vi "getValue.vi"(8 "error in (no error)":errorcluster, 11 "tBSONBoolean in":refnum<class "tBSONBoolean.lvclass">) -> (0 "error out":errorcluster, 2 "Value":bool, 3 "tBSONBoolean out":refnum<class "tBSONBoolean.lvclass">)   [LabVIEW 2013, in "BSON.lvlib" / "tBSONBoolean.lvclass"]
uses:
  tBSONBoolean.lvclass
  tBSONBoolean.lvclass/tBSONBoolean.ctl
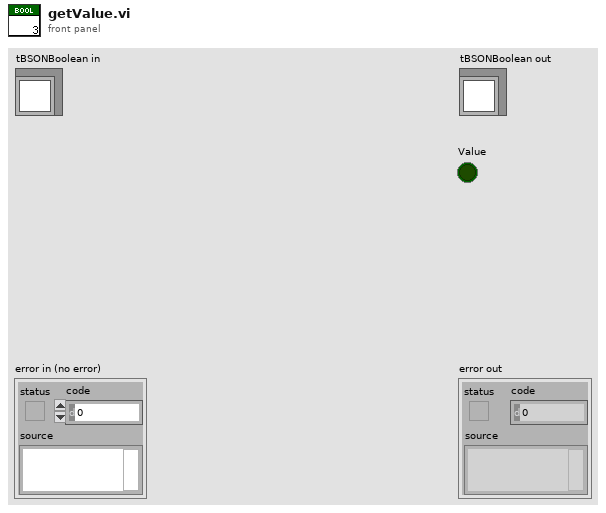
[diagram p1: front panel]
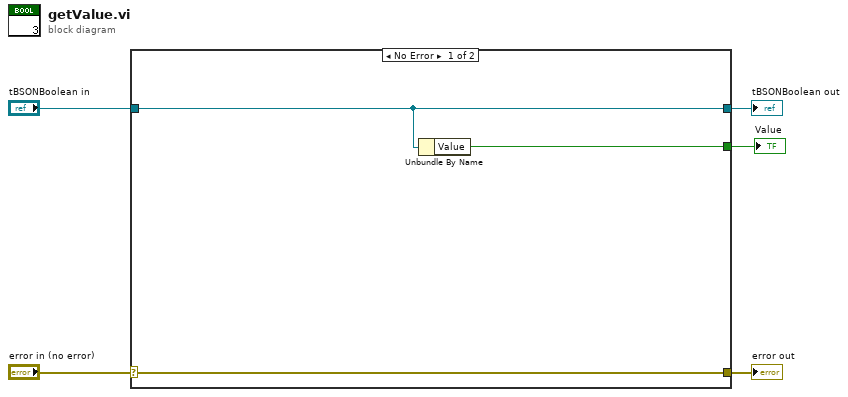
[diagram p0: block diagram]
diagram:
  n1 = case shown="No Error" "error in (no error)" {
    selector: "error in (no error)" -> [w8 w10]
    tunnel: [w8 w10] -> w4
    tunnel: [w7 w9] -> w2
    tunnel: "tBSONBoolean in" -> [w7 w9]
    tunnel: [w6 _] -> w1
    frame No Error {
      n2 = Unbundle By Name(w7) -> ("Value"=w6:bool)
    }
    frame Error {
    }
  }
  "error out" <- w4
  "tBSONBoolean out" <- w2
  "Value" <- w1
